vi "Synchronized AO test.vi"() -> ()   [LabVIEW 2021]
uses:
  <instrlib>/niScope/Controls/niScope trigger source.ctl
  <vilib>/userdefined/High Color/nirio_resource_hc.ctl
  <instrlib>/niScope/Controls/niScope input clock source.ctl
  5785_3.2GHz_one channel/5785_3.2GHz_one channel.lvclass
  pulse_tx_vis/emitter params.ctl
  pulse_tx_vis/mode_type.ctl
  <instrlib>/niScope/Controls/niScope trigger coupling.ctl
  <instrlib>/niScope/Controls/niScope trigger slope.ctl
  <instrlib>/niScope/Utility/niScope Get Channel Name From String.vi
  <instrlib>/niScope/Configure/Trigger/niScope Configure Trigger Immediate.vi
  <instrlib>/niScope/Configure/Trigger/niScope Configure Trigger Edge.vi
  <instrlib>/niScope/Configure/Trigger/niScope Configure Trigger Digital.vi
  <instrlib>/niScope/Configure/Trigger/niScope Configure Trigger Window.vi
  <instrlib>/niScope/Configure/Trigger/niScope Configure Trigger Hysteresis.vi
  <instrlib>/niScope/Acquire/Fetch/niScope Multi Fetch WDT.vi
  <vilib>/Analysis/NI_AALBase.lvlib
  <resource>/objmgr/sessionReference.rc
panel:
  in  "Bitfile path":path=path "C:/Users/PXIe8108_Demo/Documents/CHAIM DATA/chaim/5785_sync_for_elbit/tx_pulse/pulse Tx Folder_lv_21/TDMS files/pulses.tdms"
  in  "devicess":T1[](array[typedef])=["IF_transceiver_0", "IF_transceiver_1", "IF_transceiver_2"]
  out "Waveform(s) 3":dbl[](graph)=[-0.0] caption="skew"
  out "f for test":dbl=500000000.0
  out "histogram ch 1-2":T2(graph)={"X Values"=[-0.0, -0.0, -0.0, -0.0, -0.0, -0.0, -0.0, -0.0, -0.0, -0.0], "Histogram: h(x)"=[0, 0, 0, 0, 0, 0, 0, 0, 0, 1]}
  out "histogram ch 1-3":T2(graph)={"X Values"=[-0.0, -0.0, -0.0, -0.0, -0.0, -0.0, -0.0, -0.0, -0.0, -0.0], "Histogram: h(x)"=[0, 0, 0, 0, 0, 0, 0, 0, 0, 1]}
  out "max-min 1 - 2":dbl format="%#_6p"
  out "max-min 1-3":dbl format="%#_6p"
  out "Waveform(s) 2":dbl[](graph)=[-0.0] caption="skew"
  in  "frequency test":dbl=500000000.0 format="%#_6p"
  out "Actual Skew [s] 2":dbl=-0.0 format="%#_6p"
  out "error out":errorcluster={"status"=TRUE, "code"=-250032, "source"="niTClk Configure For Homogeneous Triggers.vi:2010001<append>\nSession index (starts at zero): 0"}
  in  "stop":bool
  out "Actual Iteration":i32=1
  out "Actual Skew [s]":dbl=-0.0 format="%#_6p"
  in  "Number of Iterations":i32=100
  in  "Vertical Range":dbl=1.0 caption="Vertical Range (V)" format="%.2f"
  in  "Min Record Length":i32=6400000 caption="Min. Record Length" format="%.1p"
  out "Waveform(s)":waveform(dbl)[](graph)
  out "Actual Record Length":i32
  out "Actual Sample Rate":dbl format="%#.2p"
  in  "Vertical Offset":dbl caption="Vertical Offset (V)" format="%.2p"
  in  "Trigger Delay":dbl caption="Trigger Delay (s)" format="%#.4p"
  in  "Reference Position":dbl caption="Ref Position" format="%.1f"
  in  "Trigger Type":T3(tab)=enum."Hysteresis"
  in  "Trigger Level":dbl=0.1 format="%.2f"
  in  "trigger source 2":T4="0" caption="trigger source"
  in  "Trigger Slope 2":enum16{"Positive", "Negative"}(ring) caption="Trigger Slope"
  in  "Trigger Source 2":string(combo)="VAL_PFI_1" caption="Trigger Source"
  in  "Coupling 2":T5(ring)=enum."DC" caption="Trigger Coupling"
  in  "High Level":dbl=0.1 caption="Window High Level" format="%.2f"
  in  "Low Level":dbl=-0.1 caption="Window Low Level" format="%.2f"
  in  "Window Mode":enum16{"Entering", "Leaving"}(ring)
  in  "Trigger Source 3":string(combo)="0" caption="Trigger Source"
  in  "Hysteresis":dbl=0.05 format="%.2f"
  in  "Trigger Source 4":string(combo)="0" caption="Trigger Source"
  in  "Trigger Level 2":dbl caption="Trigger Level" format="%.2f"
  in  "Coupling 3":T5(ring)=enum."DC" caption="Trigger Coupling"
  in  "Trigger Slope 3":enum16{"Positive", "Negative"}(ring) caption="Trigger Slope"
  in  "Resource Name":refnum<k15>="PXI1Slot10" caption="Resource Name(s)"
  # "Aquisition"
  # "Results"
  # "Note: When configured for Immediate reference trigger, this example does not configure any additional trigger settings - the acquisition is triggered as soon as possible after being initiated by driver software."
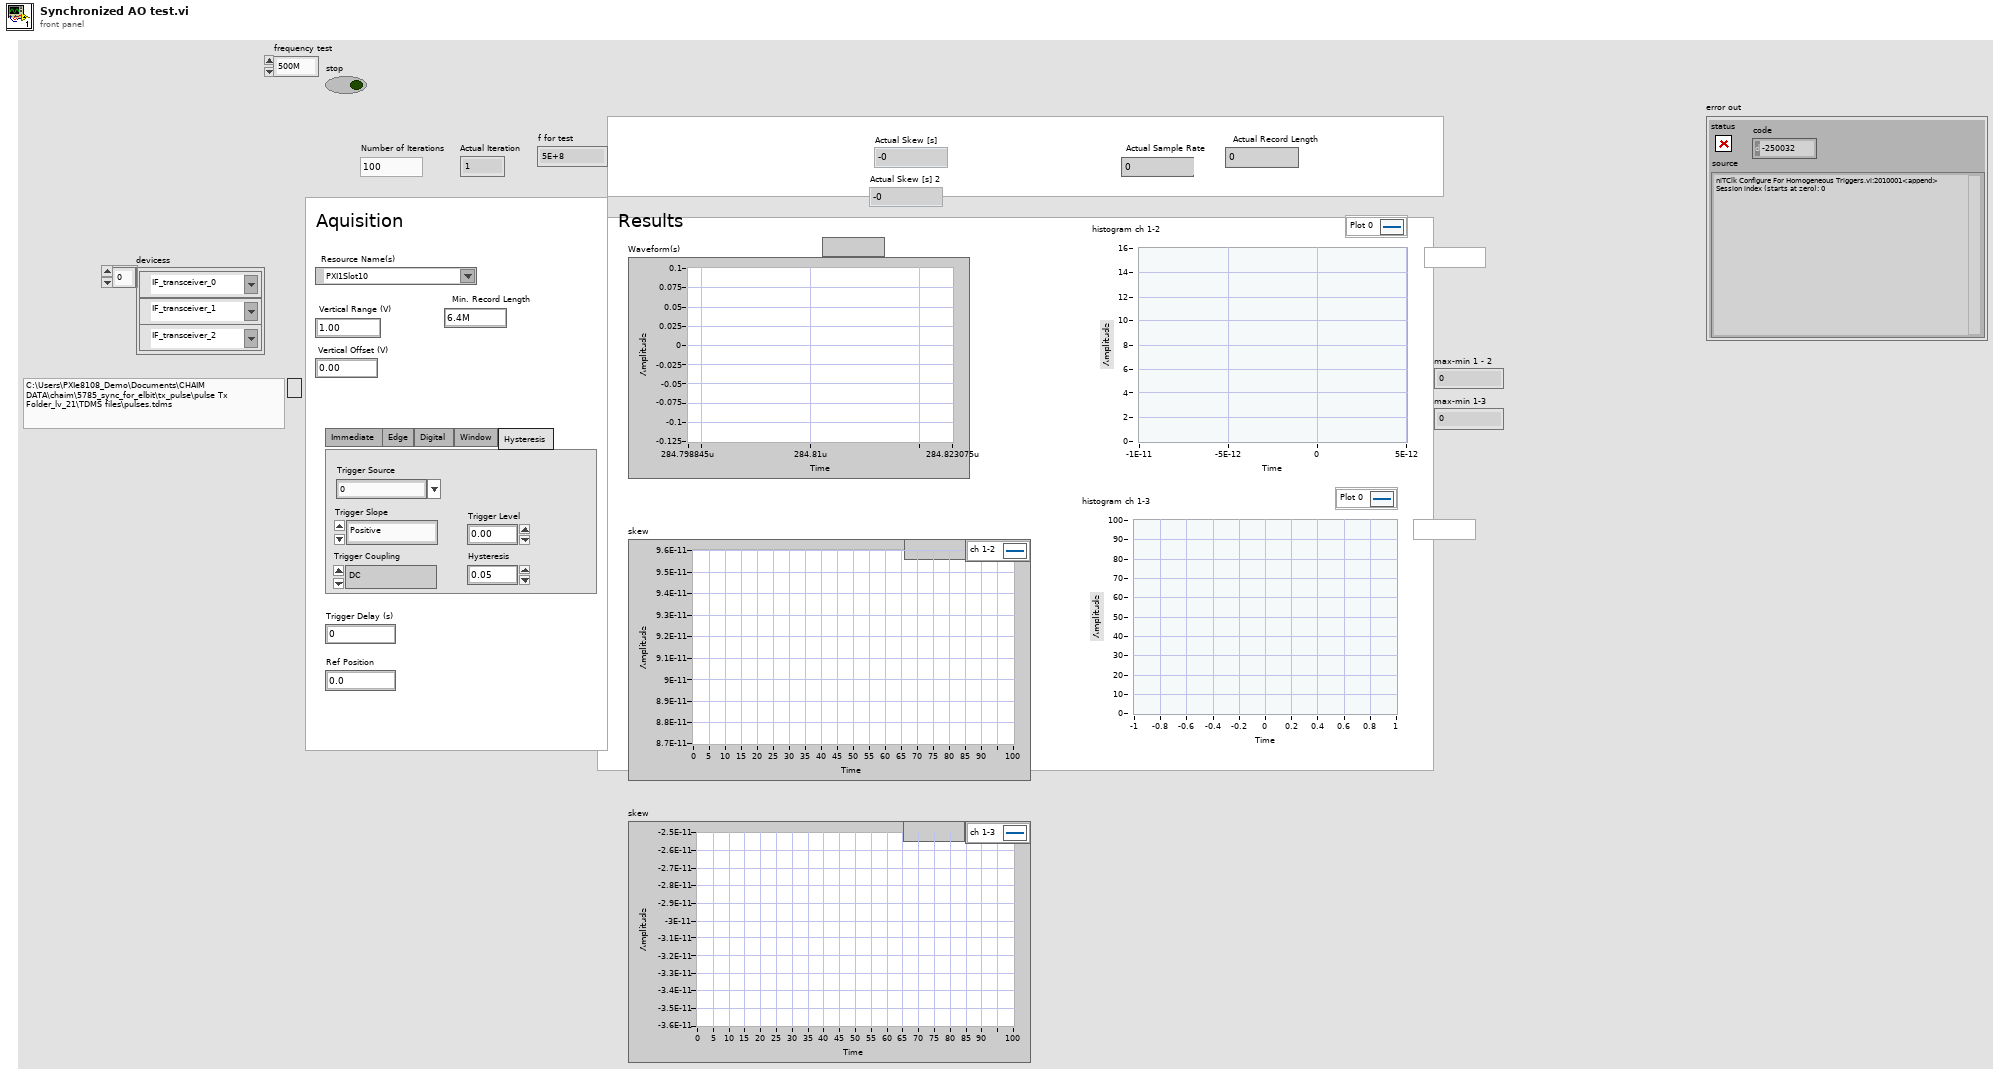
[diagram p1: front panel]
types:
  T1 = typedef "nirio_resource_hc.ctl" = tag
  T2 = cluster{"X Values":dbl[], "Histogram: h(x)":i32[]}
  T3 = enum32{"Immediate", "Edge", "Digital", "Window", "Hysteresis"}
  T4 = typedef "niScope trigger source.ctl" = string
  T5 = enum16{"AC", "DC", "HF Reject", "LF Reject", "AC Plus HF Reject"}
  T6 = typedef "mode_type.ctl" = enum8{"CW", "NC - CW", "NC - cw", "LFM", "BPSK", "QPSK"}
  T7 = typedef "emitter params.ctl" = cluster{"f set":dbl[], "hop rate (Hz)":dbl, "d.c.":dbl, "amp (dB)":dbl, "mod type":T6, "mod depth":dbl, "DOA":dbl, "t start":dbl, "t end":dbl}
  T8 = cluster{"vst_device":refnum<k15>[], "RF gain ":dbl, "buffer size":u32, "center frequency (Hz) ":dbl, "P2P sample rate":dbl, "mode":enum16{"USRP - 180MHz", "5785 - 2*180MHz", "5785 - 3.2GHz", "P2P - VST"}, "devicess":T1[], "file paths":path[], "gen for df":bool}
  T9 = typedef "niScope input clock source.ctl" = u16
  T10 = typedef "niScope trigger slope.ctl" = i32
  T11 = typedef "niScope trigger coupling.ctl" = u16
  T12 = typedef "PDW_lv2.ctl" = cluster{"t start":dbl, "frequency (Hz)":dbl, "duration (sec)":dbl, "amp (lin)":dbl, "mod type":T6, "mod depth":dbl, "phase (rad)":dbl[]}
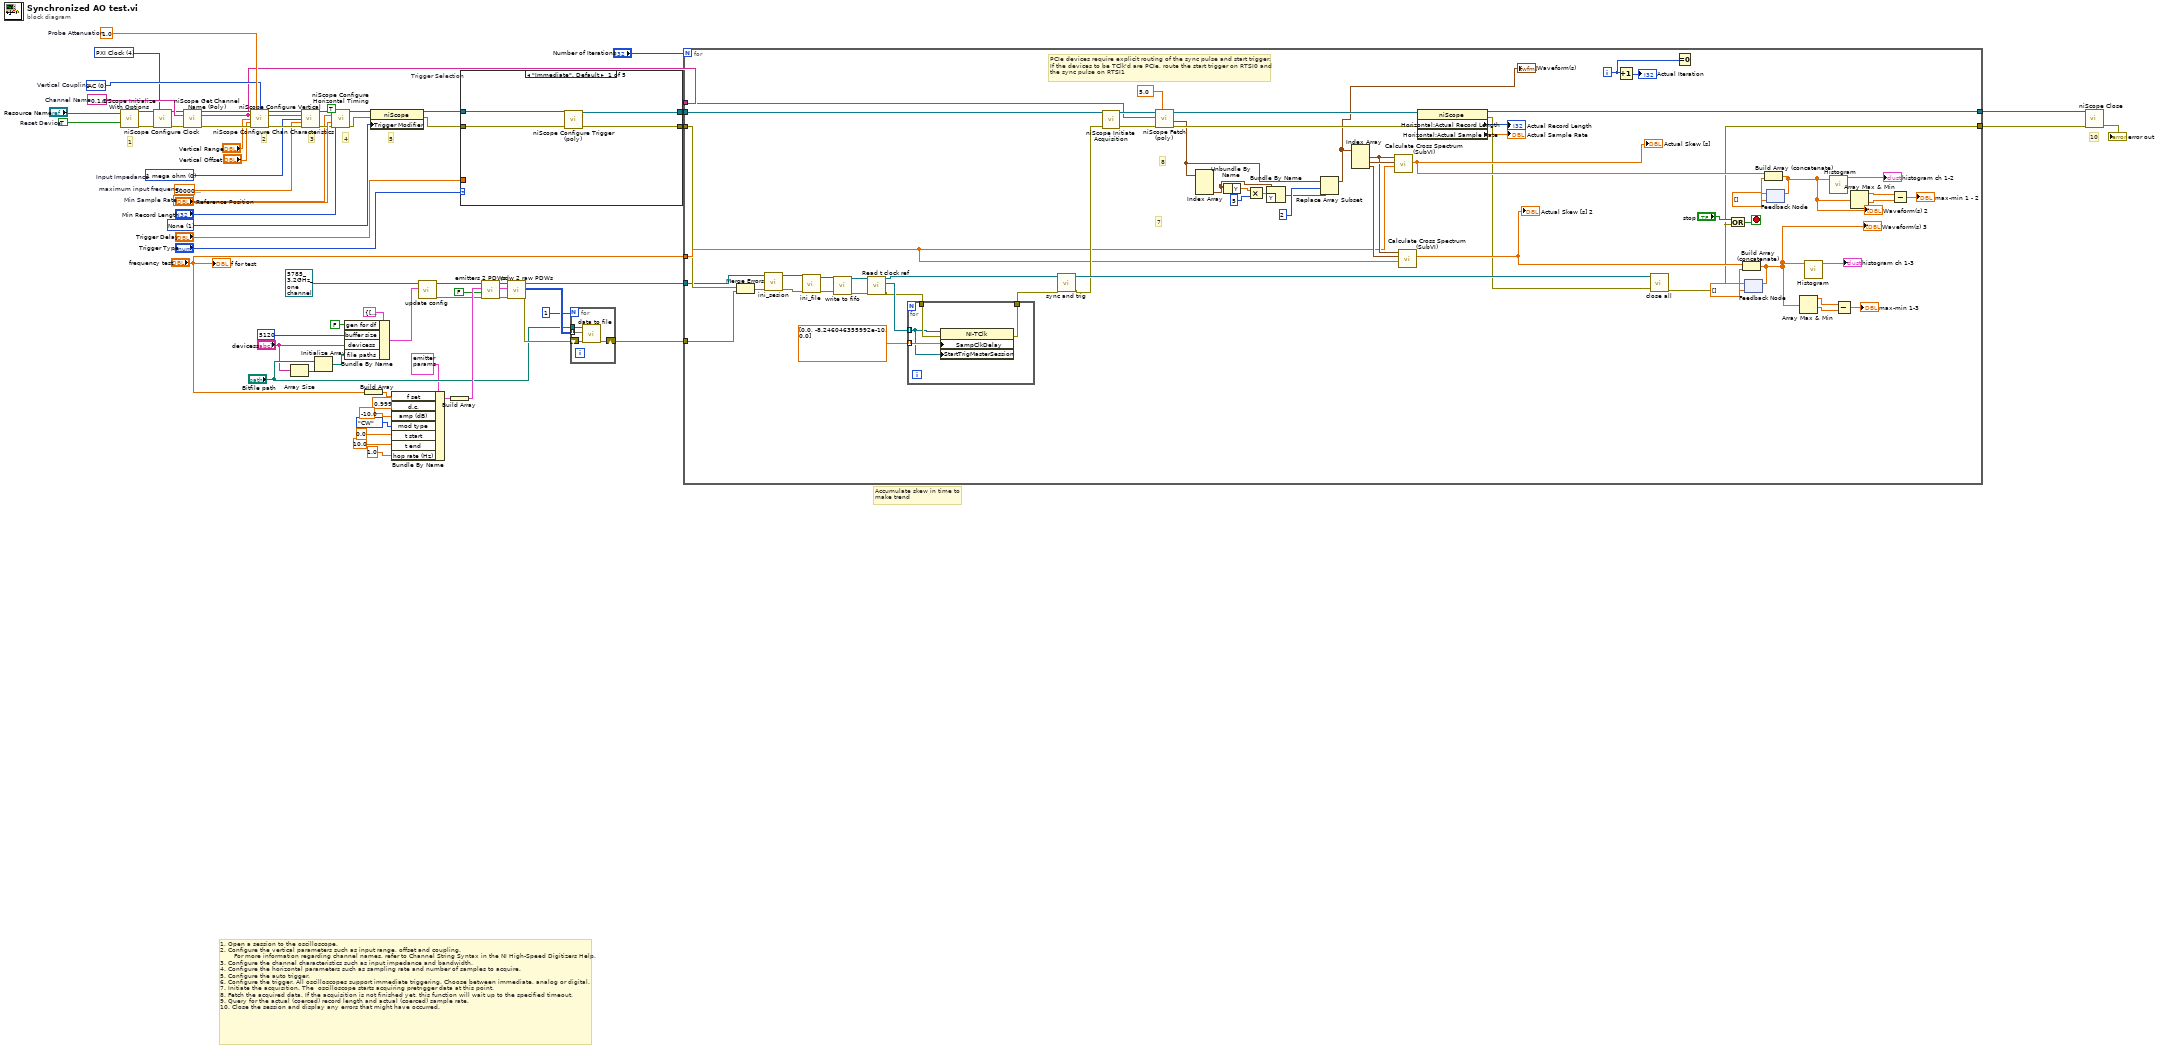
[diagram p0: block diagram]
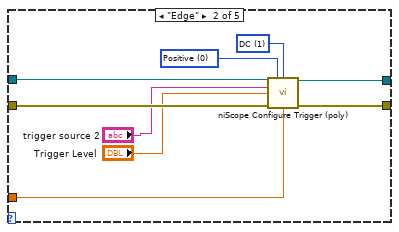
[diagram p2: hidden frame]
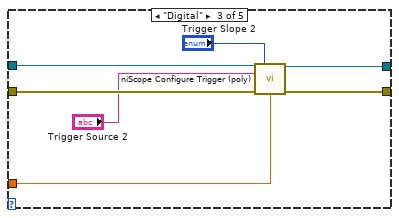
[diagram p3: hidden frame]
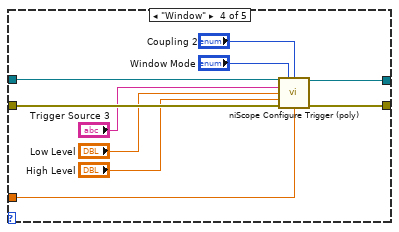
[diagram p4: hidden frame]
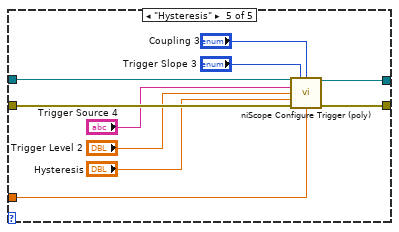
[diagram p5: hidden frame]
diagram:
  w33 = 300000000.0  # maximum input frequency
  w34 = T9 4 items=["None"=0, "RTSI Clock"=1, "PFI 0"=6, "PFI 1"=2, "PFI 2"=3, "PXI Clock"=4, "External"=5, "Clock In"=7] ("input clock source")
  w49 = 1 items=["None"=1, "Auto Trigger"=2] ("Triggering:Trigger Modifier")
  w38 = 1250000000.0  # Min Sample Rate
  w46 = u32 0 items=["1 mega ohm"=0, "50 ohms"=2]  # Input Impedance
  w47 = 0 items=["AC", "DC", "Ground"]  # Vertical Coupling
  w48 = 1.0  # Probe Attenuation
  w50 = "0,1,2"  # Channel Name
  w44 = TRUE  # Reset Device
  # "Accumulate skew in time to\nmake trend"
  # "10"
  # "5"
  # "2"
  # "3"
  # "4"
  # "1. Open a session to the oscilloscope.\n2. Configure the vertical parameters such as input range, offset and coupling.\n       For more information regarding channel names, refer to Channel String Syntax in the NI High-Speed Digitizers Help.\n3. Configure the channel characteristics such as input impedance and bandwidth.\n4. Configure the horizontal parameters such as sampling rate and number of samples to acquire.\n5. Configure the auto trigger.\n6. Configure the trigger. All oscilloscopes support immediate triggering. Choose between immediate, analog or digital.\n7. Initiate the acquisition. The  oscilloscope starts acquiring pretrigger data at this point.\n8. Fetch the acquired data. If the acquisition is not finished yet, this function will wait up to the specified timeout.\n9. Query for the actual (coerced) record length and actual (coerced) sample rate.\n10. Close the session and display any errors that might have occurred."
  # "1"
  n1 = call <instrlib>:"niScope Initialize With Options.vi"("resource name"="Resource Name", "reset device"=w44) -> ("instrument handle"=w68:refnum<k15>, "error out"=w36:errorcluster)  [unwired: 12 in]
  n2 = call <instrlib>:"niScope Configure Clock.vi"("instrument handle"=w68, "input clock source"=w34, "error in"=w36) -> ("instrument handle out"=w37:refnum<k15>, "error out"=w35:errorcluster)  [unwired: 11 in]
  n3 = call-poly <instrlib>:"niScope Get Channel Name (Poly).vi"("instrument handle"=w37, "index"=w50, "error in"=w35) -> ("instrument handle out"=w66:refnum<k15>, "channel name"=w43:string, "error out"=w67:errorcluster)  [unwired: 10 in]
  n4 = call <instrlib>:"niScope Configure Vertical.vi"("instrument handle"=w66, "probe attenuation"=w48, "vertical coupling"=w47, "channels"=w43, "vertical range"="Vertical Range", "vertical offset"="Vertical Offset", "error in"=w67) -> ("instrument handle out"=w54:refnum<k15>, "error out"=w55:errorcluster)  [unwired: 7 in]
  n5 = Array Size(array="devicess") -> (size(s)=w18:i32)
  n6 = call <instrlib>:"niScope Configure Chan Characteristics.vi"("instrument handle"=w54, "channels"=w43, "input impedance"=w46, "maximum input frequency"=w33, "error in"=w55) -> ("instrument handle out"=w57:refnum<k15>, "error out"=w56:errorcluster)  [unwired: 9 in]
  n7 = Initialize Array("Bitfile path", w18) -> (w20:path[])
  n8 = call <instrlib>:"niScope Configure Horizontal Timing.vi"("instrument handle"=w57, "enforce realtime"=TRUE ("Enforce Realtime"), "min sample rate"=w38, "reference position"="Reference Position", "error in"=w56, "min record length"="Min Record Length") -> ("instrument handle out"=w61:refnum<k15>, "error out"=w62:errorcluster)  [unwired: 8 in]
  n9 = Bundle By Name(cluster=T8 {"vst_device"=["VST_1"], "RF gain "=10.0, "buffer size"=100288, "center frequency (Hz) "=1600000000.0, "P2P sample rate"=1250000000.0, "mode"=enum."5785 - 3.2GHz", "devicess"=["IF_transceiver_0", "IF_transceiver_1", "IF_transceiver_2"], "file paths"=[path "C:/Users/PXIe8108_Demo/Documents/CHAIM DATA/chaim/5785_sync_for_elbit/data/pdw_test_file.tdms", path "C:/Users/PXIe8108_Demo/Documents/CHAIM DATA/chaim/5785_sync_for_elbit/data/pdw_test_file_1.tdms", path "C:/Users/PXIe8108_Demo/Documents/CHAIM DATA/chaim/5785_sync_for_elbit/data/pdw_test_file_2.tdms", path "C:/Users/PXIe8108_Demo/Documents/CHAIM DATA/chaim/5785_sync_for_elbit/data/pdw_test_file_3.tdms", path "C:/Users/PXIe8108_Demo/Documents/CHAIM DATA/chaim/5785_sync_for_elbit/data/pdw_test_file_4.tdms"], "gen for df"=TRUE} ("user configurations"), "gen for df"=FALSE, "buffer size"=u32 5120, "devicess"="devicess", "file paths"=w20) -> (w17:T8)
  n10 = Build Array("frequency test") -> (w31:dbl[])
  n11 = property on="Property Node" class="niScope"(reference=w61, error in=w62, "Trigger Modifier"=w49) -> (reference out=w64:refnum<k15>, error out=w63:errorcluster)
  n12 = Bundle By Name(cluster=T7 {"f set"=[], "hop rate (Hz)"=0.0, "d.c."=0.0, "amp (dB)"=0.0, "mod type"=enum."CW", "mod depth"=0.0, "DOA"=0.0, "t start"=0.0, "t end"=0.0} ("Cluster"), "f set"=w31, "d.c."=0.999, "amp (dB)"=-10.0, "mod type"=mode_type."CW", "t start"=0.0, "t end"=10.0, "hop rate (Hz)"=1.0) -> (w29:T7)
  n13 = call-dynamic "update config.vi"("user configurations"=w17, "5785_3.2GHz_one channel in"=refnum<class "5785_3.2GHz_one channel.lvclass"> refnum ("5785_3.2GHz_one channel.lvclass")) -> ("error out"=w25:errorcluster, "5785_3.2GHz_one channel out"=w24:refnum<class "5785_3.2GHz_one channel.lvclass">)  [unwired: 6 in, 2 out]
  n14 = Build Array(w29) -> (w30:T7[])
  n15 = case "Trigger Selection" shown="\"Immediate\", Default" "Trigger Type" {
    tunnel: w63 -> [w73 w82 w89 w99 w109]
    tunnel: [w70 w78 w85 w95 w105] -> w32
    tunnel: w64 -> [w72 w81 w88 w98 w108]
    tunnel: [w71 w79 w86 w96 w107] -> w42
    tunnel: "Trigger Delay" -> [_ w80 w87 w97 w106]
    frame "Immediate", Default {
      n16 = call-poly <instrlib>:"niScope Configure Trigger (poly).vi"("instrument handle"=w72, "error in"=w73) -> ("instrument handle out"=w71:refnum<k15>, "error out"=w70:errorcluster)  [unwired: 12 in]
    }
    frame "Edge" {
      w74 = T10 0 items=["Positive", "Negative"] ("trigger slope")
      w76 = T11 1 items=["AC"=0, "DC"=1, "HF Reject"=3, "LF Reject"=4, "AC Plus HF Reject"=1001] ("trigger coupling")
      n17 = call-poly <instrlib>:"niScope Configure Trigger (poly).vi"("instrument handle"=w81, "trigger slope"=w74, "trigger coupling"=w76, "trigger source"="trigger source 2", "trigger level"="Trigger Level", "error in"=w82, "trigger delay"=w80) -> ("instrument handle out"=w79:refnum<k15>, "error out"=w78:errorcluster)  [unwired: 7 in]
    }
    frame "Digital" {
      n18 = call-poly <instrlib>:"niScope Configure Trigger (poly).vi"("instrument handle"=w88, "trigger slope"="Trigger Slope 2", "trigger source"="Trigger Source 2", "error in"=w89, "trigger delay"=w87) -> ("instrument handle out"=w86:refnum<k15>, "error out"=w85:errorcluster)  [unwired: 9 in]
    }
    frame "Window" {
      n19 = call-poly <instrlib>:"niScope Configure Trigger (poly).vi"("instrument handle"=w98, "trigger window mode"="Window Mode", "trigger coupling"="Coupling 2", "trigger source"="Trigger Source 3", "low level"="Low Level", "high level"="High Level", "error in"=w99, "trigger delay"=w97) -> ("instrument handle out"=w96:refnum<k15>, "error out"=w95:errorcluster)  [unwired: 6 in]
    }
    frame "Hysteresis" {
      n20 = call-poly <instrlib>:"niScope Configure Trigger (poly).vi"("instrument handle"=w108, "trigger slope"="Trigger Slope 3", "trigger coupling"="Coupling 3", "trigger source"="Trigger Source 4", "trigger level"="Trigger Level 2", "hysteresis"="Hysteresis", "error in"=w109, "trigger delay"=w106) -> ("instrument handle out"=w107:refnum<k15>, "error out"=w105:errorcluster)  [unwired: 6 in]
    }
  }
  n21 = call-dynamic "emitters 2 PDWs.vi"("error in (no error)"=w25, "random startinig phase"=FALSE, "emmiter"=w30, "device_type in"=w24) -> ("error out"=w23:errorcluster, "sorted PDWs"=w22:T12[], "device_type out"=w21:refnum<class "5785_3.2GHz_one channel.lvclass">)  [unwired: 5 in]
  n22 = call-dynamic "pdw 2 raw PDWs.vi"("error in (no error)"=w23, "PDWs"=w22, "device_type in"=w21) -> ("error out"=w27:errorcluster, "Array"=w28:u64[][], "device_type out"=w2:refnum<class "5785_3.2GHz_one channel.lvclass">)  [unwired: 6 in]
  n23 = for {
    N: 1 -> [_]
    tunnel: "Bitfile path" -> [w113]
    tunnel: w28 -> [w110] mode=indexing
    shift-right: [w111] -> w3
    shift-left: w27 -> [w112]
    n24 = call "data to file.vi"("error in (no error)"=w112, "Array"=w110, "Path"=w113) -> ("error out"=w111:errorcluster)  [unwired: 8 in]
  }
  n25 = for {
    N: "Number of Iterations" -> [_]
    tunnel: w43 -> [w167]
    tunnel: w42 -> [w166]
    tunnel: [w165] -> w40
    tunnel: [w126] -> w39
    tunnel: w32 -> [w119]
    tunnel: "frequency test" -> [w120]
    tunnel: w3 -> [w116]
    tunnel: w2 -> [w118]
    i -> [w158]
    stop <- w164 stop-if-true
    # "7"
    # "8"
    # "PCIe devices require explicit routing of the sync pulse and start trigger.\nIf the devices to be TClk'd are PCIe, route the start trigger on RTSI0 and\nthe sync pulse on RTSI1"
    n26 = Merge Errors(w119, w116) -> (w115:errorcluster)
    n27 = call-dynamic "ini_sesion.vi"("error in (no error)"=w115, "5785_3.2GHz_one channel in"=w118) -> ("error out"=w114:errorcluster, "5785_3.2GHz_one channel out"=w117:refnum<class "5785_3.2GHz_one channel.lvclass">)  [unwired: 8 in]
    n28 = call-dynamic "ini_file.vi"("device_type in"=w117, "error in (no error)"=w114) -> ("device_type out"=w132:refnum<class "5785_3.2GHz_one channel.lvclass">, "error out"=w131:errorcluster)  [unwired: 11 in, 1 out]
    n29 = call-dynamic "write to fifo.vi"("5785_3.2GHz_one channel in"=w132, "error in (no error)"=w131) -> ("5785_3.2GHz_one channel out"=w130:refnum<class "5785_3.2GHz_one channel.lvclass">, "error out"=w128:errorcluster)  [unwired: 9 in, 3 out]
    n30 = call-dynamic "Read t clock ref.vi"("error in (no error)"=w128, "5785_3.2GHz_one channel in"=w130) -> ("error out"=w122:errorcluster, "t clock ref"=w129:refnum<k20>[], "5785_3.2GHz_one channel out"=w121:refnum<class "5785_3.2GHz_one channel.lvclass">)  [unwired: 7 in]
    n31 = for {
      tunnel: w129 -> [w175] mode=indexing
      tunnel: dbl[] [0.0, -8.246046355992e-10, 0.0] -> [w178] mode=indexing
      tunnel: w122 -> [w177]
      tunnel: [w176] -> w124
      n32 = property class="NI-TClk"(reference=w175, error in=w177, "SampClkDelay"=w178, "StartTrigMasterSession"=w175) -> (error out=w176:errorcluster)  [unwired: 1 out]
    }
    n33 = call-dynamic "sync and trig.vi"("error in (no error)"=w124, "5785_3.2GHz_one channel in"=w121) -> ("error out"=w123:errorcluster, "5785_3.2GHz_one channel out"=w127:refnum<class "5785_3.2GHz_one channel.lvclass">)  [unwired: 8 in]
    n34 = call <instrlib>:"niScope Initiate Acquisition.vi"("instrument handle"=w166, "error in"=w123) -> ("instrument handle out"=w173:refnum<k15>, "error out"=w163:errorcluster)  [unwired: 12 in]
    n35 = call-poly <instrlib>:"niScope Fetch (poly).vi"("timeout"=5.0 ("Timeout (s)"), "error in"=w163, "channels"=w167, "instrument handle"=w173) -> ("error out"=w171:errorcluster, "wfm"=w135:waveform(dbl)[], "instrument handle out"=w172:refnum<k15>)  [unwired: 4 in, 1 out]
    n36 = Index Array(array=w135) -> (element #3=w133:waveform(dbl))  [unwired: 3 in, 2 out]
    n37 = Unbundle By Name(w133) -> ("Y"=w140:dbl[])
    n38 = Multiply(x=w140, y=5) -> (x*y=w137:dbl[])
    n39 = Bundle By Name(cluster=w133, "Y"=w137) -> (w136:waveform(dbl))
    n40 = Replace Array Subset(array=w135, new element=w136, index=2) -> (w134:waveform(dbl)[])
    "Waveform(s)" <- w134
    n41 = Index Array(array=w134) -> (element #1=w160:waveform(dbl), element #2=w168:waveform(dbl), element #3=w161:waveform(dbl))  [unwired: 3 in]
    n42 = call "Calculate Cross Spectrum (SubVI).vi"("Center Frequency (Hz)"=w120, "signal in 2"=w168, "signal in 1"=w160) -> ("Skew [s]"=w150:dbl)  [unwired: 7 in, 1 out]
    "Actual Skew [s]" <- w150
    n43 = call "Calculate Cross Spectrum (SubVI).vi"("Center Frequency (Hz)"=w120, "signal in 2"=w161, "signal in 1"=w160) -> ("Skew [s]"=w157:dbl)  [unwired: 7 in, 1 out]
    "Actual Skew [s] 2" <- w157
    n44 = property class="niScope"(reference=w172, error in=w171) -> (reference out=w165:refnum<k15>, error out=w125:errorcluster, "Horizontal:Actual Record Length"=→"Actual Record Length":i32, "Horizontal:Actual Sample Rate"=→"Actual Sample Rate":dbl)
    n45 = Increment(x=w158) -> (x+1=→"Actual Iteration":i32)
    n46 = call-dynamic "close all.vi"("error in (no error)"=w125, "5785_3.2GHz_one channel in"=w127) -> ("error out"=w126:errorcluster)  [unwired: 8 in, 1 out]
    n47 = Equal To 0?(x=w158) -> ()  [unwired: 1 out]
    n48 = Or(x="stop", y=w126) -> (x .or. y?=w164:bool)
    n49 = feedback #1(dbl[] []) -> (w156:dbl[])
    n50 = Build Array (concatenate)(w157, w156) -> (w142:dbl[])
    "Waveform(s) 3" <- w142
    n51 = feedback-in #1(w142) -> ()
    n52 = feedback #2(dbl[] []) -> (w151:dbl[])
    n53 = Build Array (concatenate)(w150, w151) -> (w143:dbl[])
    "Waveform(s) 2" <- w143
    n54 = feedback-in #2(w143) -> ()
    n55 = Array Max & Min(array=w142) -> (max value=w152:dbl, min value=w153:dbl)  [unwired: 2 out]
    n56 = call <vilib>:"Histogram.vi"("X"=w142) -> ("Histogram Graph"=→"histogram ch 1-3":T2)  [unwired: 7 in, 3 out]
    n57 = call <vilib>:"Histogram.vi"("X"=w143) -> ("Histogram Graph"=→"histogram ch 1-2":T2)  [unwired: 7 in, 3 out]
    n58 = Subtract(x=w152, y=w153) -> (x-y=→"max-min 1-3":dbl)
    n59 = Array Max & Min(array=w143) -> (max value=w148:dbl, min value=w147:dbl)  [unwired: 2 out]
    n60 = Subtract(x=w148, y=w147) -> (x-y=→"max-min 1 - 2":dbl)
  }
  n61 = call <instrlib>:"niScope Close.vi"("instrument handle"=w40, "error in"=w39) -> ("error out"=→"error out":errorcluster)  [unwired: 13 in]
  "f for test" <- "frequency test"
